vi "Read Experiment Configuration.vi"(8 "error in (no error)":errorcluster, 11 "Control Experiment in":refnum<class "Control Experiment.lvclass">) -> (0 "error out":errorcluster, 2 "Experiment Description":T1={"User"="", "Device"="", "Device Path"=path "", "Device Description"="", "Experiment Path"=path "", "Experiment Description"="", "Instrument"=enum."MNK", "Instruments"=[], "Sweep"=[{"key"="OFF", "value"=variant}, {"key"="OFF", "value"=variant}, {"key"="OFF", "value"=variant}, {"key"="OFF", "value"=variant}]}, 3 "Control Experiment out":refnum<class "Control Experiment.lvclass">)   [LabVIEW 2019, in "Control Experiment.lvclass"]
uses:
  Control Experiment.lvclass
  Typedefs/Experiment Description--cluster.ctl
  Typedefs/Instrument--enum.ctl
  Typedefs/Instrument Types--combo.ctl
  Control Experiment.lvclass/Control Experiment.ctl
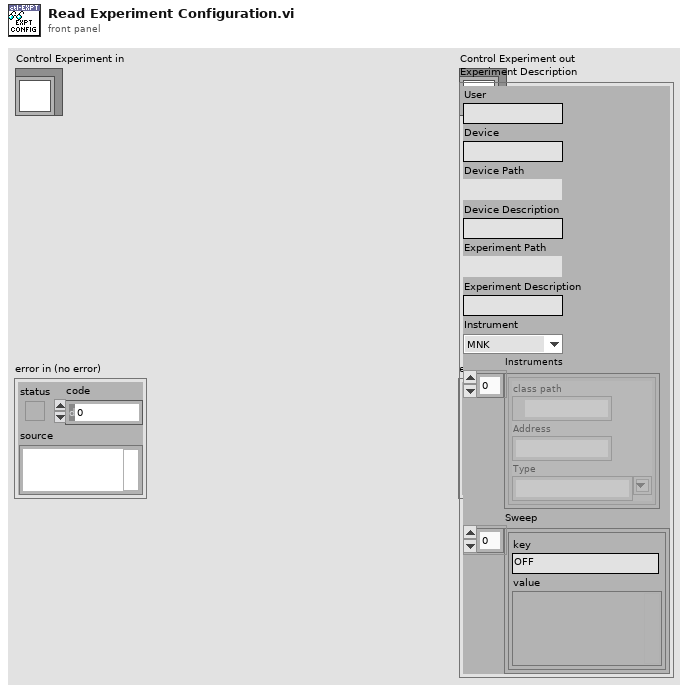
[diagram p1: front panel]
types:
  T1 = typedef "Control Experiment.lvclass/Experiment Description--cluster.ctl" = cluster{"User":string, "Device":string, "Device Path":path, "Device Description":string, "Experiment Path":path, "Experiment Description":string, "Instrument":T2, "Instruments":cluster{"class path":path, "Address":string, "Type":T3}[], "Sweep":cluster{"key":string, "value":variant}[]}
  T2 = typedef "Control Experiment.lvclass/Instrument--enum.ctl" = enum16{"----- AFM/EBL -----", "AGILENT", "CYPHER", "Gemini2", "JEOL", "MFP3D", "----- Cryostat -----", "CF900", "DR200", "MNK", "PPMS (simulated)", "PPMS 1", "PPMS 2", "PPMS 3", "----- Optics -----", "THz 1 (Element 2/Montana)", "THz 2 (Tsunami/Janis)"}
  T3 = typedef "Control Experiment.lvclass/Instrument Types--combo.ctl" = string
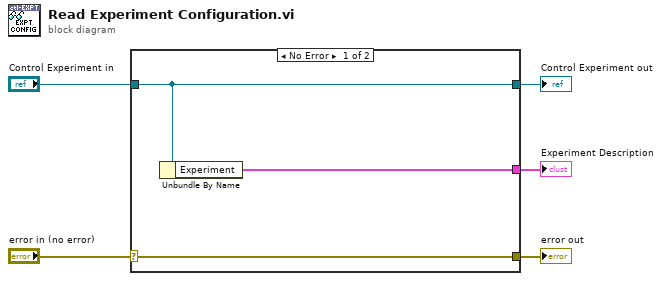
[diagram p0: block diagram]
diagram:
  n1 = case shown="No Error" "error in (no error)" {
    selector: "error in (no error)" -> [w8 w9]
    tunnel: [w8 w9] -> w4
    tunnel: [w7 w10] -> w2
    tunnel: "Control Experiment in" -> [w7 w10]
    tunnel: [w6 _] -> w1
    frame No Error {
      n2 = Unbundle By Name(w7) -> ("Experiment"=w6:T1)
    }
    frame Error {
    }
  }
  "error out" <- w4
  "Control Experiment out" <- w2
  "Experiment Description" <- w1
